vi "Test@ShowCMD__Parameter.vi"(1 "ParamterIn":string) -> (0 "ParamterOut":string)   [LabVIEW 2020]
panel:
  in  "Parameter":string(combo)
  in  "Device":string(combo)
  in  "Confirm":bool
  # "Test@ShowCMD $ExternDevice,$Parameter"
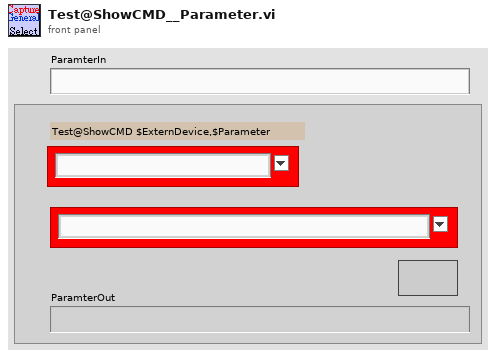
[diagram p1: front panel]
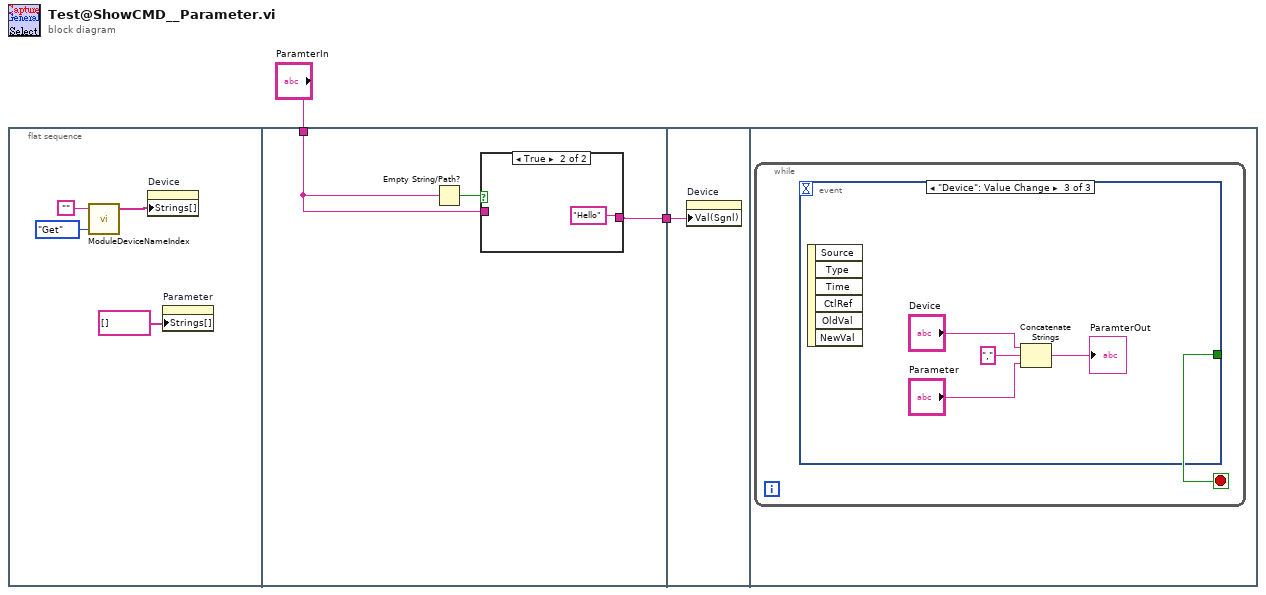
[diagram p0: block diagram]
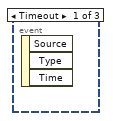
[diagram p3: hidden frame]
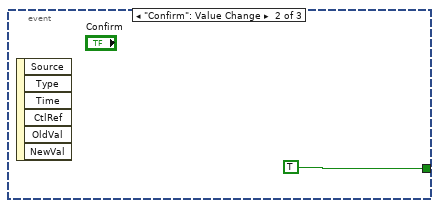
[diagram p4: hidden frame]
diagram:
  n1 = flat-sequence {
    tunnel: "ParamterIn" -> [w8]
    tunnel: [w7] -> w1
    tunnel: w1 -> [w12]
    frame #0 {
      n2 = call "ModuleDeviceNameIndex.vi"("OP"=enum16{"Get", "Update", "Init"}."Get", "DeviceName"="") -> ("DeviceList"=w5:string[])  [unwired: 1 in, 2 out]
      n3 = property on="Device" class="CmbBox"("Strings[]"=w5) -> ()  [unwired: 2 in, 2 out]
      n4 = property on="Parameter" class="CmbBox"("Strings[]"=string[] [] ("Strings []")) -> ()  [unwired: 2 in, 2 out]
    }
    frame #1 {
      n5 = Empty String/Path?(string/path=w8) -> (empty?=w9:bool)
      n6 = case shown="True" w9 {
        tunnel: w8 -> [w10 _]
        tunnel: [w10 "Hello" ("ParamterIn")] -> w7
        frame False {
        }
        frame True {
        }
      }
    }
    frame #2 {
      n7 = property on="Device" class="CmbBox"("Val(Sgnl)"=w12) -> ()  [unwired: 2 in, 2 out]
    }
    frame #3 {
      n8 = while {
        stop <- w13 stop-if-true
        n9 = event shown="[2] \"Device\": Value Change" {
          selector: _ -> [_ _ _]
          dyn-events: _ -> [_ _ _]
          timeout: _ -> [_ _ _]
          tunnel: [_ TRUE _] -> w13
          event Timeout {
            n10 = event-data() -> ()  [unwired: 1 in, 3 out]
          }
          event "Confirm": Value Change {
            n11 = event-data() -> ()  [unwired: 1 in, 6 out]
          }
          event "Device": Value Change {
            n12 = event-data() -> ()  [unwired: 1 in, 6 out]
            n13 = Concatenate Strings("Device", "," ("string"), "Parameter") -> (→"ParamterOut":string)
          }
        }
      }
    }
  }
